vi "Insight_Streaming.vi"() -> ()   [LabVIEW 2015]
panel:
  out "error out 2":errorcluster
  out "error out":errorcluster
  in  "Data Queue":refnum<queue>
  in  "stop":bool
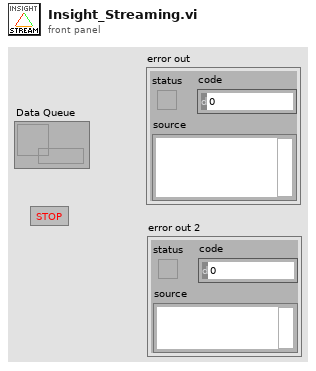
[diagram p1: front panel]
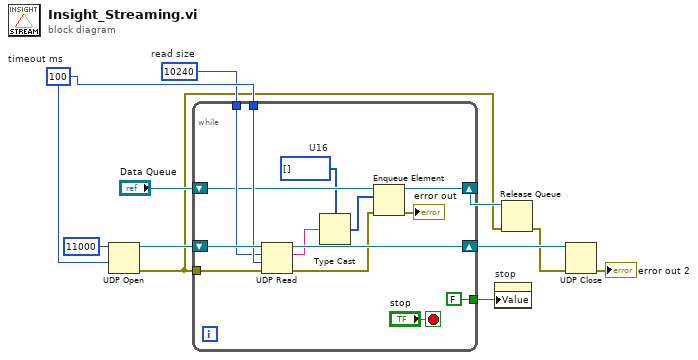
[diagram p0: block diagram]
diagram:
  w8 = 10240  # read size
  w9 = 100  # timeout ms
  n1 = UDP Open(9:w9, 11:u16 11000 ("port")) -> (port=w10:refnum<k16>, 0:w3:errorcluster)  [unwired: 3 in, 1 out]
  n2 = while {
    shift-right: [w20] -> w7
    shift-left: w10 -> [w23]
    tunnel: w9 -> [w22]
    tunnel: w8 -> [w21]
    shift-right: [w17] -> w6
    shift-left: "Data Queue" -> [w19]
    tunnel: w3 -> [w24]
    tunnel: [FALSE ("stop")] -> w1
    stop <- "stop" stop-if-true
    w14 = u16[] []  # U16
    n3 = UDP Read(connection ID=w23, max size (548)=w21, timeout ms (25000)=w22, 8:w24) -> (data out=w16:string, error out=w18:errorcluster, 3:w20:refnum<k16>)  [unwired: 2 out]
    n4 = Type Cast(type=w14, x=w16) -> (*(type *) &x=w15:u16[])
    n5 = Enqueue Element(queue=w19, element=w15, error in (no error)=w18) -> (queue out=w17:refnum<queue>, error out=→"error out":errorcluster)  [unwired: 1 in, 1 out]
  }
  n6 = property on="stop" class="Bool (strict)"("Value"=w1) -> ()  [unwired: 2 in, 2 out]
  n7 = Release Queue(queue=w6, error in (no error)=w3) -> (error out=w5:errorcluster)  [unwired: 1 in, 2 out]
  n8 = UDP Close(connection ID=w7, 8:w5) -> (error out=→"error out 2":errorcluster)  [unwired: 1 out]
